vi "Derivative Cal.vi"(8 "dt":dbl, 9 "Reinit":bool, 10 "process variable in":dbl, 11 "PID gains":T1) -> (2 "deriv Term":dbl)   [LabVIEW 2023]
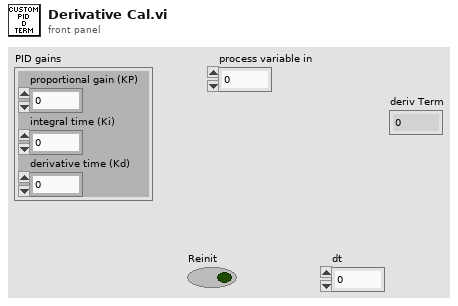
[diagram p1: front panel]
types:
  T1 = cluster{"proportional gain (KP)":dbl, "integral time (Ki)":dbl, "derivative time (Kd)":dbl}
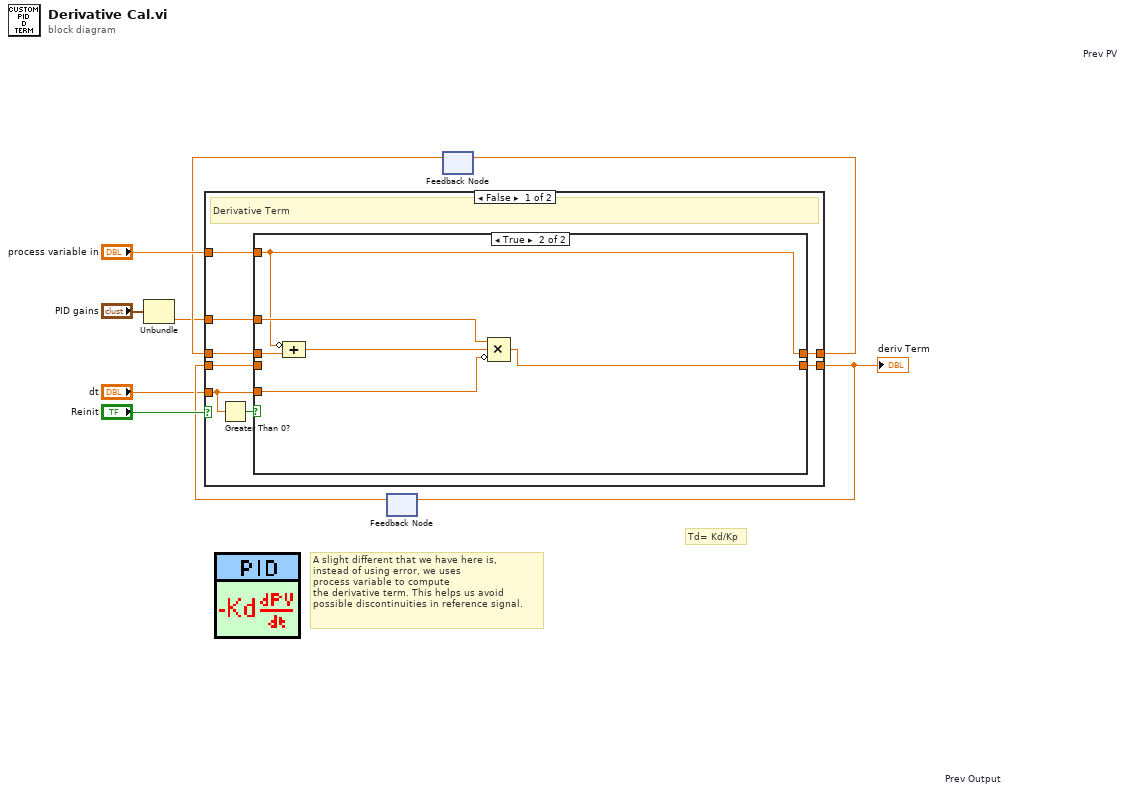
[diagram p0: block diagram]
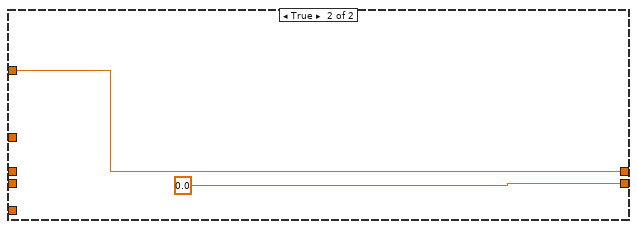
[diagram p3: hidden frame]
diagram:
  # "A slight different that we have here is, \ninstead of using error, we uses \nprocess variable to compute \nthe derivative term. This helps us avoid \npossible discontinuities in reference signal."
  # "Td= Kd/Kp"
  n1 = Unbundle("PID gains") -> ("derivative time (Kd)"=w2:dbl)  [unwired: 2 out]
  n2 = feedback #1 "Prev Output"() -> (w4:dbl)  [unwired: 1 in]
  n3 = feedback #2 "Prev PV"() -> (w3:dbl)  [unwired: 1 in]
  n4 = case shown="False" "Reinit" {
    tunnel: w3 -> [w17 _]
    tunnel: w2 -> [w14 _]
    tunnel: "process variable in" -> [w16 w27]
    tunnel: [w13 w27] -> w7
    tunnel: [w15 0.0] -> w5
    tunnel: w4 -> [w11 _]
    tunnel: "dt" -> [w10 _]
    frame False {
      # "Derivative Term"
      n5 = Greater Than 0?(x=w10) -> (x > 0?=w12:bool)
      n6 = case shown="True" w12 {
        tunnel: w17 -> [w19 w21]
        tunnel: w10 -> [_ w24]
        tunnel: w16 -> [_ w22]
        tunnel: [w18 w23] -> w15
        tunnel: w14 -> [_ w25]
        tunnel: [w19 w22] -> w13
        tunnel: w11 -> [w18 _]
        frame False {
          # "dt = 0 min"
        }
        frame True {
          n7 = Compound Arithmetic op=ADD(invert w22, w21) -> (w20:dbl)
          n8 = Compound Arithmetic op=MULTIPLY(w25, w20, invert w24) -> (w23:dbl)
        }
      }
    }
    frame True {
    }
  }
  "deriv Term" <- w5
  n9 = feedback-in #1(w5) -> ()
  n10 = feedback-in #2(w7) -> ()
